vi "ROI grp-Case-Timeout functions.vi"(8 "error in (no error)":errorcluster, 11 "ROI grouping window queue":refnum<queue>) -> (0 "error out":errorcluster)   [LabVIEW 2020]
uses:
  Globals/gl_ROI grp window globals.vi
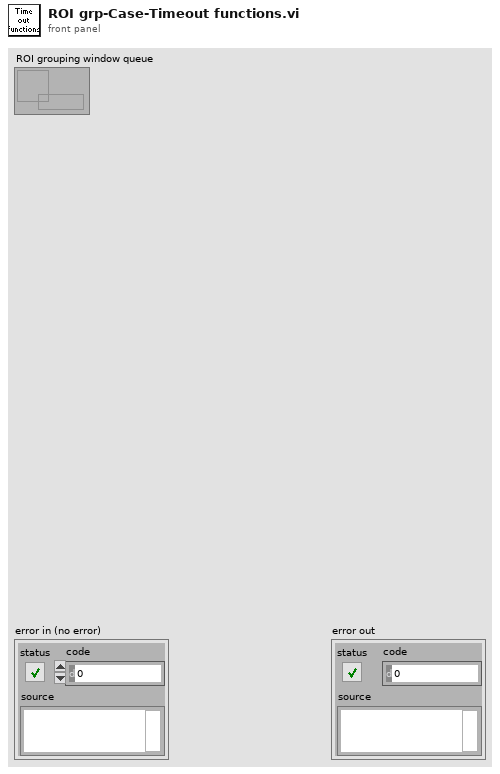
[diagram p1: front panel]
types:
  T1 = typedef "ROI grp-window ctrl refs.ctl" = cluster{"This VI":refnum<vi>, "Pane":refnum<vi>, "Table":refnum<vi>}
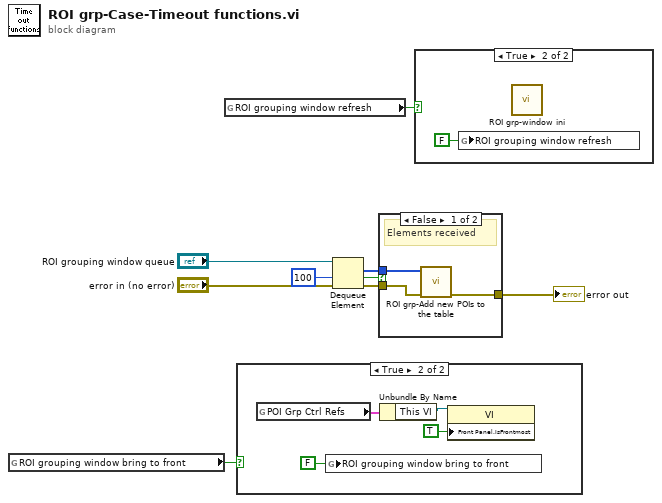
[diagram p0: block diagram]
diagram:
  n1 = global read "gl_ROI grp window globals.vi" "ROI grouping window bring to front"() -> (w7:bool)
  n2 = global read "gl_ROI grp window globals.vi" "ROI grouping window refresh"() -> (w1:bool)
  n3 = case shown="True" w7 {
    frame False {
    }
    frame True {
      n4 = global read "gl_ROI grp window globals.vi" "POI Grp Ctrl Refs"() -> (w10:T1)
      n5 = global write "gl_ROI grp window globals.vi" "ROI grouping window bring to front"(FALSE ("Bring POI grouping window to front")) -> ()
      n6 = Unbundle By Name(w10) -> ("This VI"=w12:refnum<vi>)
      n7 = property class="VI"(reference=w12, "Front Panel.IsFrontmost"=TRUE ("Front Panel Window:Is Frontmost")) -> ()  [unwired: 1 in, 2 out]
    }
  }
  n8 = Dequeue Element(queue="ROI grouping window queue", timeout in ms (-1)=100, error in (no error)="error in (no error)") -> (element=w5:i32[], timed out?=w4:bool, error out=w3:errorcluster)  [unwired: 1 out]
  n9 = case shown="False" w4 {
    tunnel: w5 -> [w16 _]
    tunnel: w3 -> [w15 w17]
    tunnel: [w14 w17] -> w2
    frame False {
      # "Elements received"
      n10 = call "ROI grp-Add new POIs to the table.vi"("error in (no error)"=w15, "New POI indexes"=w16) -> ("error out"=w14:errorcluster)  [unwired: 8 in, 1 out]
    }
    frame True {
      # "Queue timed out"
    }
  }
  "error out" <- w2
  n11 = case shown="True" w1 {
    frame False {
    }
    frame True {
      n12 = global write "gl_ROI grp window globals.vi" "ROI grouping window refresh"(FALSE ("ROI grouping window refresh")) -> ()
      n13 = call "ROI grp-window ini.vi"() -> ()  [unwired: 10 in, 2 out]
    }
  }
